vi "pressure filter.vi"(10 "Ts":dbl=1e-05, 11 "P":dbl) -> (3 "P":dbl)   [LabVIEW 2019]
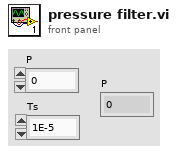
[diagram p1: front panel]
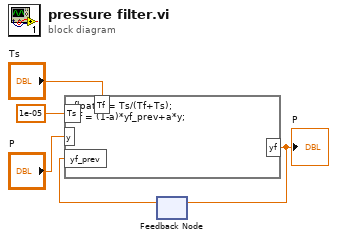
[diagram p0: block diagram]
diagram:
  n1 = feedback #1() -> (w5:dbl)  [unwired: 1 in]
  n2 = formula code="float a = Ts/(Tf+Ts);\nyf = (1-a)*yf_prev+a*y;"("Tf"="Ts", "Ts"=1e-05 ("input variable"), "y"="P", "yf_prev"=w5) -> ("yf"=w3:dbl)
  "P" <- w3
  n3 = feedback-in #1(w3) -> ()
